vi "onProcessStop.vi"(8 "error in (no error)":errorcluster, 11 "EmbeddedMainUI":refnum<class "EmbeddedMainUI.lvclass">) -> (0 "error out":errorcluster, 3 "EmbeddedMainUI out":refnum<class "EmbeddedMainUI.lvclass">)   [LabVIEW 2016, in "EmbeddedMainUI.lvclass"]
uses:
  EmbeddedMainUI.lvclass
  <vilib>/Levylab/Embedded SMO UI/EmbeddedSMO.lvclass
  C:/Program Files (x86)/National Instruments/LabVIEW 2016/vi.lib/JKI/JKI SMO/SMO/SMO.lvclass
  <vilib>/JKI/JKI SMO/SMO.UI/SMO.UI.lvclass
  <vilib>/JKI/JKI SMO/SMO/SMO.lvclass
panel:
  # "For instructions on how to use the JKI State Machine Objects, examples and video tutorials, visit:\nhttp://jki.net/state-machine-objects/\n\nJKI State Machine Objects™\nhttp://jki.net/state-machine-objects/\nCopyright (C) 2005-2015, JKI <info@jki.net>\nALL RIGHTS RESERVED"
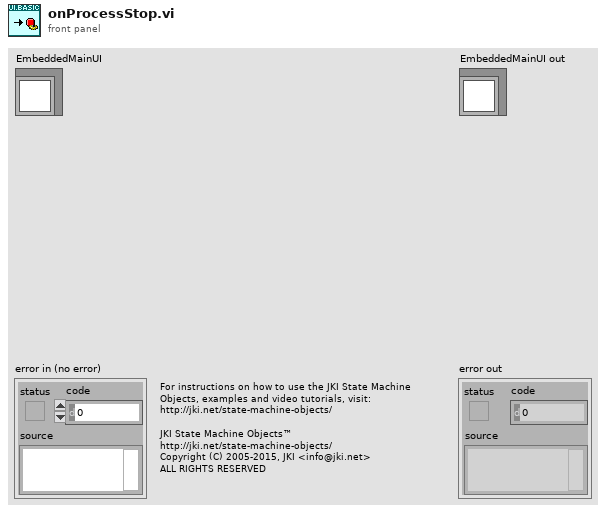
[diagram p1: front panel]
types:
  T1 = typedef "SMO.lvclass/SMOState --Enum.ctl" = enum16{"unknown", "Created", "Started", "Stopped"}
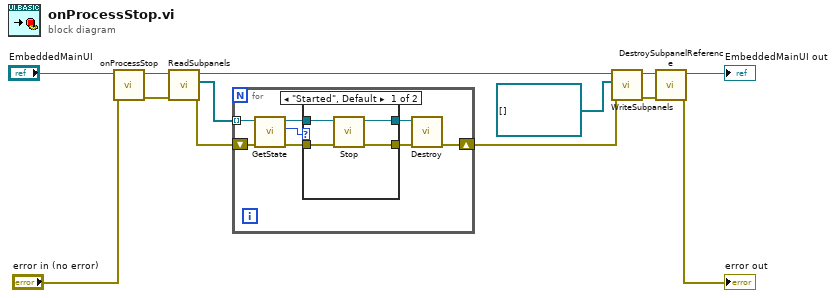
[diagram p0: block diagram]
diagram:
  n1 = call-parent "onProcessStop.vi"("error in (no error)"="error in (no error)", "SMO"="EmbeddedMainUI") -> ("error out"=w10:errorcluster, "SMO out"=w11:refnum<class "EmbeddedMainUI.lvclass">)  [unwired: 8 in]
  n2 = call "ReadSubpanels.vi"("error in (no error)"=w10, "EmbeddedMainUI in"=w11) -> ("error out"=w8:errorcluster, "Subpanels"=w9:refnum<class "EmbeddedSMO.lvclass">[], "EmbeddedMainUI out"=w7:refnum<class "EmbeddedMainUI.lvclass">)  [unwired: 7 in]
  n3 = for {
    tunnel: w9 -> [w21] mode=indexing
    shift-right: [w14] -> w6
    shift-left: w8 -> [w20]
    n4 = call <vilib>:"GetState.vi"("error in (no error)"=w20, "SMO"=w21) -> ("error out"=w17:errorcluster, "SMO State"=w19:T1, "SMO out"=w18:refnum<class "EmbeddedSMO.lvclass">)  [unwired: 7 in]
    n5 = case shown="\"Started\", Default" w19 {
      tunnel: w18 -> [w25 w27]
      tunnel: w17 -> [w24 w26]
      tunnel: [w23 w27] -> w16
      tunnel: [w22 w26] -> w15
      frame "Started", Default {
        n6 = call <vilib>:"Stop.vi"("error in (no error)"=w24, "SMO"=w25) -> ("error out"=w22:errorcluster, "SMO out"=w23:refnum<class "EmbeddedSMO.lvclass">)  [unwired: 8 in]
      }
      frame "Stopped" {
      }
    }
    n7 = call <vilib>:"Destroy.vi"("error in (no error)"=w15, "SMO"=w16) -> ("error out"=w14:errorcluster)  [unwired: 9 in]
  }
  n8 = call "WriteSubpanels.vi"("error in (no error)"=w6, "Subpanels"=refnum<class "EmbeddedSMO.lvclass">[] [], "EmbeddedMainUI in"=w7) -> ("error out"=w2:errorcluster, "EmbeddedMainUI out"=w4:refnum<class "EmbeddedMainUI.lvclass">)  [unwired: 7 in]
  n9 = call "DestroySubpanelReference.vi"("error in (no error)"=w2, "EmbeddedMainUI in"=w4) -> ("error out"=→"error out":errorcluster, "EmbeddedMainUI out"=→"EmbeddedMainUI out":refnum<class "EmbeddedMainUI.lvclass">)  [unwired: 8 in]
